vi "main.vi"() -> ()   [LabVIEW 2009]
uses:
  Support Files/VelocityState.ctl
  Support Files/TimeRec.ctl
  Support Files/LocalPose.ctl
  SimClass/Simulator.lvclass
  cRIO/Functional Global Variables/Actions for FG's.ctl
panel:
  out "Current Pose":T1={"Initial Location"={"x"=0.0, "y"=0.0}, "Initial Heading\n(degs from north)"=45.0, "Initial Location ( GPS )"={"Latitude"=0.0, "Longitude"=0.0}} {"Initial Location ( GPS )"."Longitude" format="%#_10g"; "Initial Location ( GPS )"."Latitude" format="%#_10g"}
  out "LocalPose":T2
  out "Last Yaw":dbl
  out "VelocityState":T4
  out "Current Location ( GPS )":cluster{"Latitude":dbl, "Longitude":dbl} {"Longitude" format="%#_10g"; "Latitude" format="%#_10g"}
  out "error":dbl
  in  "Loop Iteration Minimum Time":u32=100
  out "Waveform Graph":dbl[](graph)
  in  "Threshold":u32=250
  out "Turning Radius":dbl=31000000000.0
  out "Speed":dbl=133.33333333333334
  out "Compass Reading":dbl=303.2011334759296
  in  "PAUSE":bool
  out "XY Graph":cluster{dbl[], dbl[]}[](graph)=[{[35.0, 400.0, 300.0, 100.0, 300.0, 900.0, 300.0, 400.0, 500.0, 600.0, 700.0, 800.0, 200.0, 650.0, 900.0, 900.0, 800.0, 600.0], [401.0, 500.0, 0.0, 250.0, 100.0, 250.0, -400.0, 0.0, 0.0, 0.0, 0.0, 0.0, 400.0, 400.0, 400.0, 550.0, 700.0, 800.0]}, {[250.87088056783944], [819.9620618916982]}, {[250.87088056783944, 167.19553247645274], [819.9620618916982, 874.7200395916212]}, {[415.14481366760845, 410.73878540090254, 406.28405982170926, 401.781993882594, 397.23395895645433, 392.6413404187865, 388.00553722568674, 383.32796148771575, 378.6100380397561, 373.85320400699345, 369.05890836715463, 364.22861150913513, 359.3637847881498, 354.46591007754466, 349.53647931740335, 344.5769940600877, 339.58896501285085, 334.5739115776606, 329.5333613883754, 324.4688498454117, 319.38191964804645, 314.27412032449604, 309.1470077599148, 304.0021437224573, 298.84109538754876, 293.66543486050836, 288.47673869767016, 283.27658742614955, 278.0665650623987, 272.8482586297003, 267.6232576747447, 262.3931537834384, 257.15954009609175, 251.92401082213325, 246.68816075449737, 241.4535847838356, 236.221877412697, 230.99463226982752, 225.77344162473517, 220.5598959026693, 215.35558320016145, 210.16208880127624, 204.98099469471802, 199.8138790919421, 194.66231594641602, 189.5278744741782, 184.41211867583957, 179.3166068601737, 174.242891169441, 169.19251710659108, 164.1670230644875, 159.16793985729856, 154.1967902541964, 149.25508851550677, 144.3443399314505, 139.46604036361785, 134.6216757893143, 129.8127218489177, 125.04064339638354, 120.3068940530367, 115.61291576478402, 110.9601383628837, 106.34997912840475, 101.78384236050971, 97.26311894869116, 92.78918594909359, 88.36340616504867, 83.98712773195203, 79.66168370660847, 75.3883916611696, 71.16855328178877, 67.00345397211476, 62.894362461745544, 58.84253041976086, 54.84919207345166, 50.915563832362665, 47.04284391776184, 43.232211997651234, 39.484828827428146, 35.801835896307665, 32.184355079614875, 28.633488297049666, 25.15031717703215, 21.735902727227653, 18.391285011353773, 15.11748283236679, 11.915493422124541, 8.786292137619654, 5.7308321638766415, 2.7500442236024867, -0.15516370632070675, -2.983906671414104, -5.735323009167871, -8.408574611511938, -11.002847180111928, -13.517350474412183, -15.951318552350585, -18.304010003672317, -20.57470817577024, -22.762721391984428, -24.86738316229338, -26.88805238633364, -28.824113548684863, -30.674976906361906, -32.44007866845641, -34.11888116787253, -35.710873025106196, -37.21556930401573, -38.63251165953807, -39.96126847730574, -41.20143500511983, -42.35263347624249, -43.41451322446733, -44.386750790936276, -45.26905002266858, -46.06114216277109, -46.76278593230472, -47.37376760378038, -47.89390106626212, -48.32302788205874, -48.66101733498493, -48.90776647017941, -49.06320012546507, -49.12727095424492, -49.09995943992374, -48.981273901853456, -48.77125049279863, -48.46995318792426, -48.07747376530813, -47.593931777984324, -47.01947451752653, -46.354276969181, -45.59854175856486, -44.75249908994442, -43.816406676112194, -42.79054965988564, -41.675240527249514, -40.470819012169954, -39.17765199310793, -37.79613338126455, -36.32668400059214, -34.76975145960694, -33.125810015043214, -31.395360427390187, -29.57892980835561, -27.677071460302045, -25.69036470770618, -23.619414720690486, -21.46485233068256, -19.22733383825846, -16.90754081322592, -14.50617988701299, -12.023982537420181, -9.461704865805757, -6.820127366769839, -4.100054690408314, -1.3023153972081616, 1.5722382943395985, 4.522730767333968, 7.548263273185796, 10.647914205384552, 13.820739380229583, 17.06577232443655, 20.382024569535446, 23.76848595296707, 27.224124925788658, 30.747888866893675, 34.33870440365001, 37.99547773886033, 41.717094983942616, 45.50242249823208, 49.350307234298384, 53.259577089175764, 57.22904126139636, 61.25749061372028, 65.3436980414505, 69.48641884622035, 73.68439111514141, 77.93633610519373, 82.24095863274403], [1070.9881061658584, 1073.8168491309518, 1076.5682654687055, 1079.2415170710497, 1081.8357896396496, 1084.3502929339497, 1086.7842610118882, 1089.13695246321, 1091.4076506353078, 1093.5956638515222, 1095.700325621831, 1097.7209948458712, 1099.6570560082225, 1101.5079193658996, 1103.273021127994, 1104.9518236274102, 1106.5438154846438, 1108.0485117635533, 1109.4654541190757, 1110.7942109368435, 1112.0343774646576, 1113.1855759357802, 1114.247455684005, 1115.219693250474, 1116.1019924822062, 1116.8940846223086, 1117.5957283918424, 1118.206710063318, 1118.7268435257997, 1119.1559703415965, 1119.4939597945227, 1119.7407089297171, 1119.8961425850027, 1119.9602134137826, 1119.9329018994613, 1119.8142163613911, 1119.6041929523362, 1119.3028956474618, 1118.910416224846, 1118.426874237522, 1117.8524169770642, 1117.1872194287187, 1116.4314842181025, 1115.585441549482, 1114.6493491356498, 1113.6234921194232, 1112.5081829867872, 1111.3037614717077, 1110.0105944526456, 1108.6290758408022, 1107.1596264601299, 1105.6026939191447, 1103.958752474581, 1102.2283028869278, 1100.4118722678932, 1098.5100139198398, 1096.523307167244, 1094.452357180228, 1092.2977947902202, 1090.060276297796, 1087.7404832727636, 1085.3391223465505, 1082.8569249969578, 1080.2946473253435, 1077.6530698263075, 1074.932997149946, 1072.1352578567457, 1069.2607041651981, 1066.3102116922037, 1063.284679186352, 1060.1850282541532, 1057.0122030793082, 1053.767170135101, 1050.4509178900023, 1047.0644565065707, 1043.608817533749, 1040.085053592644, 1036.4942380558875, 1032.8374647206774, 1029.115847475595, 1025.3305199613055, 1021.4826352252394, 1017.5733653703619, 1013.6039011981413, 1009.5754518458173, 1005.4892444180872, 1001.3465236133172, 997.1485513443963, 992.8966063543439, 988.5919838267937, 984.2359949914672, 979.8299667247613, 975.375241145568, 970.8731752064527, 966.3251402803131, 961.7325217426453, 957.0967185495455, 952.4191428115746, 947.7012193636149, 942.9443853308522, 938.1500896910135, 933.3197928329939, 928.4549661120086, 923.5570914014035, 918.6276606412621, 913.6681753839465, 908.6801463367096, 903.6650929015195, 898.6245427122342, 893.5600311692705, 888.4731009719053, 883.3653016483548, 878.2381890837736, 873.0933250463161, 867.9322767114076, 862.7566161843672, 857.567920021529, 852.3677687500084, 847.1577463862575, 841.9394399535591, 836.7144389986036, 831.484335107297, 826.2507214199507, 821.015192145992, 815.7793420783562, 810.5447661076944, 805.3130587365558, 800.0858135936862, 794.8646229485939, 789.6510772265282, 784.4467645240202, 779.253270125135, 774.0721760185768, 768.9050604158009, 763.7534972702748, 758.619055798037, 753.5032999996984, 748.4077881840325, 743.3340724932998, 738.2836984304498, 733.2582043883464, 728.2591211811573, 723.2879715780552, 718.3462698393655, 713.4355212553093, 708.5572216874766, 703.7128571131732, 698.9039031727765, 694.1318247202423, 689.3980753768956, 684.7040970886428, 680.0513196867425, 675.4411604522635, 670.8750236843684, 666.3543002725498, 661.8803672729524, 657.4545874889075, 653.0783090558108, 648.7528650304673, 644.4795729850284, 640.2597346056475, 636.0946352959735, 631.9855437856044, 627.9337117436196, 623.9403733973105, 620.0067451562215, 616.1340252416206, 612.3233933215101, 608.5760101512868, 604.8930172201665, 601.2755364034737, 597.7246696209086, 594.2414985008909, 590.8270840510864, 587.4824663352126, 584.2086641562256, 581.0066747459833, 577.8774734614784, 574.8220134877355, 571.8412255474612]}, {[0.0, 8.258239109063283, 17.6635679516302, 28.26928085134969, 39.161034112875655, 49.351545961474756, 58.68782493571467, 67.017866895006, 74.17725616254506, 79.93157593985106, 86.00734524231453, 94.48319360575078, 105.64436487028703, 119.79167725592882, 136.94358299068747, 150.1794196360733, 164.84512081171752, 180.911713938689, 198.27358070071088, 216.77350429907193, 235.8092408864332, 255.1902209511005, 272.62384059728083, 290.25086600452346, 307.9346913572528, 325.5367474666883, 342.87942162910025, 360.2220957915122, 376.0280427586526, 391.9430716500898, 407.9108111753572, 422.5728055023587, 437.47556231438506, 452.5412559123831, 467.6519786813084, 482.6778140366067, 497.95146078225406, 513.8552236079469, 530.3377967718476, 547.0991140448708, 564.116287401357, 581.5716748487926, 599.3034974177289, 617.2698170600805, 635.4402994256407, 653.6804251256779, 671.7908807905975, 689.9856022328188, 706.4126193604907, 723.1005733700046, 739.963298873506, 756.8529674826408, 773.5504360275042, 789.8403344502048, 805.3515380864515, 819.6617215096924, 832.3140886250497, 843.200174463986, 852.4303276119743, 859.4839933491301, 863.7335964441816, 864.7675329350542, 863.7568239435701, 860.3907306643073, 854.3479289558276, 845.4083990435004, 837.0746902438183, 826.973110391912, 814.9603185789508, 800.9883210595851, 784.9800736112029, 767.0818857558896, 747.6182647298988, 732.8362291802346, 717.1776661256229, 700.7226353767547, 683.5753213617098, 665.8647841032133, 647.8264266153427, 629.7231234483743, 611.5363362750118, 596.2012632718238, 580.4652358635182, 564.408396193986, 548.1917784471037, 531.961267905226, 515.876775330523, 500.2101580493559, 485.16185522372234, 474.0051421448708, 462.8484290660192, 451.69171598716764, 440.5350029083161, 429.3782898294645, 418.22157675061294, 407.0648636717614, 395.9081505929098, 384.75143751405824, 373.5947244352067, 362.4380113563551, 351.28129827750354, 340.12458519865197, 328.9678721198004, 317.81115904094884, 306.65444596209727, 295.4977328832457, 284.34101980439414, 273.18430672554257, 262.027593646691, 250.87088056783944], [0.0, 12.328596362905685, 24.313045923484637, 35.865186506569145, 47.75528456479064, 60.89370394730574, 75.29412013383347, 90.99290161882688, 108.06433194829125, 126.50346678912352, 145.814740377611, 165.3810317097952, 184.94444001419743, 204.165762572179, 222.3316303279354, 233.66288031356822, 244.11977587242683, 253.48717156117036, 261.52322332137487, 267.99720891922806, 273.6281558953824, 278.324449702282, 280.84890240628783, 281.82999720091664, 281.24981789324136, 279.1025398162905, 275.40458966575017, 271.70663951520976, 269.7061592666714, 268.97013199980813, 268.86835635614165, 268.2364589423116, 266.480429242474, 263.5329284594952, 259.3377937103711, 253.85256193168433, 248.2881210338638, 243.92967377612416, 240.85675779555444, 237.71946831793488, 234.54566810056866, 232.8429787662082, 232.6828200848, 233.3175442229486, 233.95948113539436, 235.4416482831041, 238.60310931659052, 241.77529872967, 244.56280159826372, 248.87479650382113, 254.85314881697008, 262.63920115244434, 272.35045410822636, 284.111807811969, 297.9244947604338, 313.6561633759146, 330.9617022784776, 349.83474276684797, 371.0198243205319, 394.5080390795776, 419.86008534092036, 439.5780549826773, 460.26950127953415, 481.79548414219704, 503.8942815691288, 526.0232330481643, 541.7200682960488, 557.1819167795918, 572.2488388431018, 586.617354269714, 600.0202190589248, 612.0278146679726, 622.2118716284103, 628.2397295487174, 633.1902346453021, 636.9208635631228, 639.2929552421908, 640.1761610137296, 639.460294815211, 637.0847932487015, 634.7022118498005, 633.9962228687847, 634.4960528781803, 636.2942836022781, 639.4678027745167, 644.0782427338557, 650.1687764225292, 657.7069481835645, 666.6397243319143, 673.9407880252373, 681.2418517185604, 688.5429154118834, 695.8439791052065, 703.1450427985295, 710.4461064918526, 717.7471701851756, 725.0482338784986, 732.3492975718217, 739.6503612651447, 746.9514249584678, 754.2524886517908, 761.5535523451139, 768.8546160384369, 776.15567973176, 783.456743425083, 790.757807118406, 798.0588708117291, 805.3599345050521, 812.6609981983752, 819.9620618916982]}]
  in  "LIDAR Characteristics":T5={"Num of Sectors"=180, "Field of View (Degs)"=180.0, "Max Range"=300.0}
  in  "Obstacle Radius":dbl=30.0
  in  "Initial Vehicle Pose":T1={"Initial Location"={"x"=0.0, "y"=0.0}, "Initial Heading\n(degs from north)"=45.0, "Initial Location ( GPS )"={"Latitude"=0.0, "Longitude"=0.0}} {"Initial Location ( GPS )"."Longitude" format="%#_10g"; "Initial Location ( GPS )"."Latitude" format="%#_10g"}
  in  "stop":bool
  in  "Timestep (s)":dbl=0.1
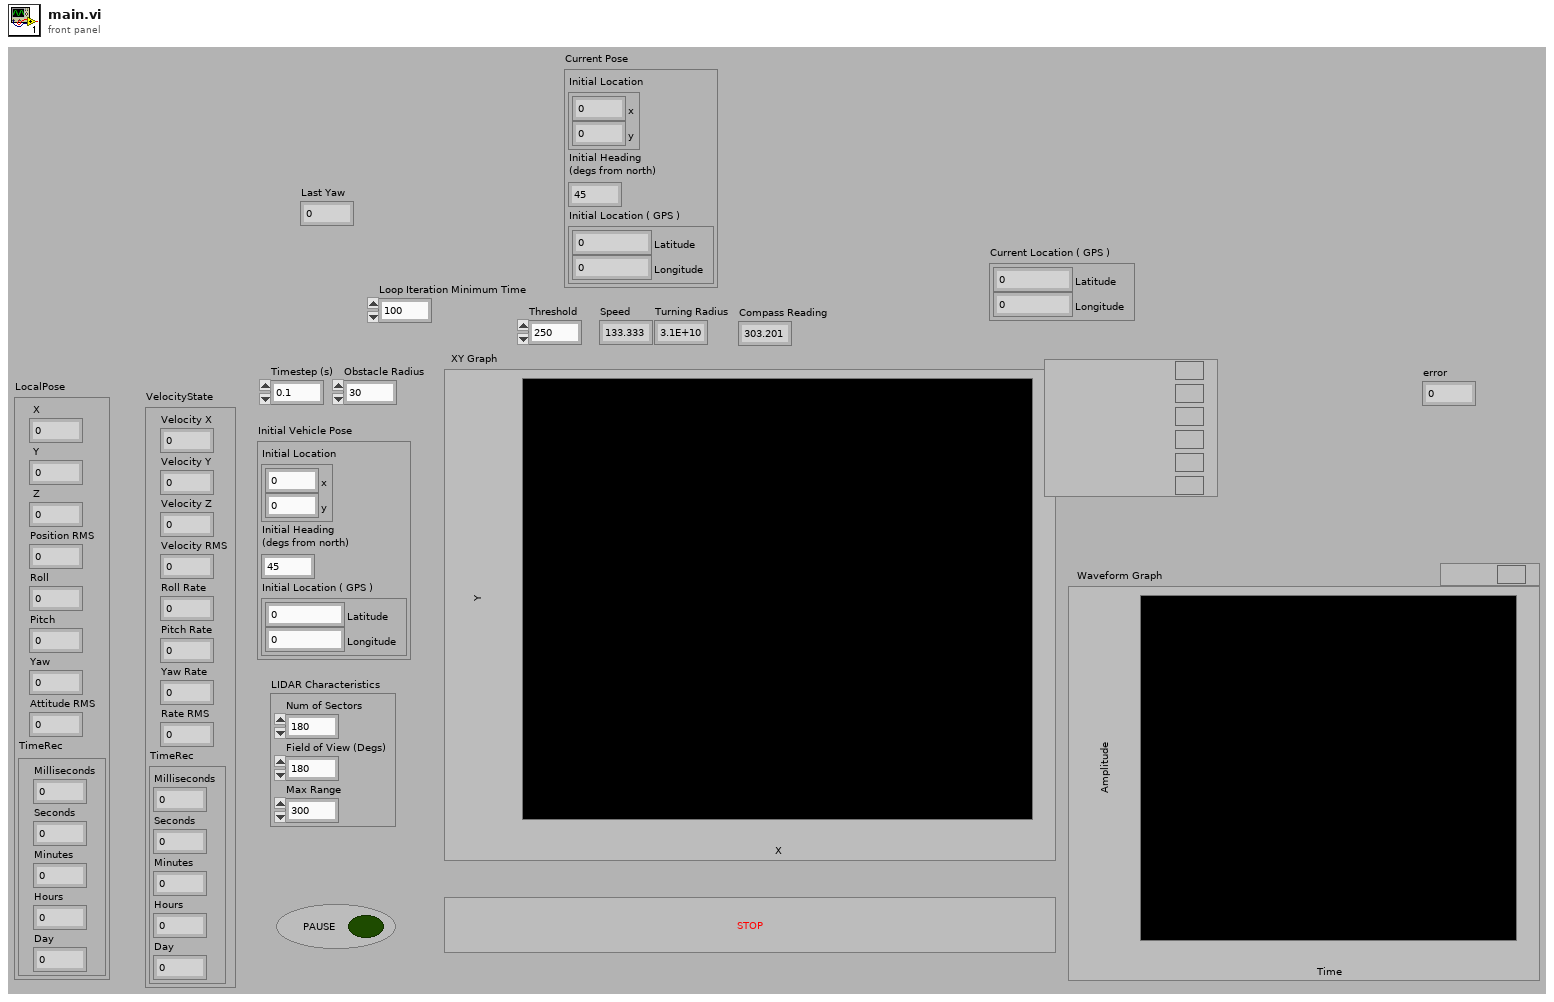
[diagram p1: front panel]
types:
  T1 = cluster{"Initial Location":cluster{"x":dbl, "y":dbl}, "Initial Heading\n(degs from north)":dbl, "Initial Location ( GPS )":cluster{"Latitude":dbl, "Longitude":dbl}}
  T2 = typedef "LocalPose.ctl" = cluster{" X":dbl, " Y":dbl, " Z":dbl, "Position RMS":dbl, "Roll":dbl, "Pitch":dbl, "Yaw":dbl, "Attitude RMS":dbl, "TimeRec":T3}
  T3 = typedef "TimeRec.ctl" = cluster{"Milliseconds":u32, "Seconds":u32, "Minutes":u32, "Hours":u32, "Day":u32}
  T4 = typedef "VelocityState.ctl" = cluster{"Velocity X":dbl, "Velocity Y":dbl, "Velocity Z":dbl, "Velocity RMS":dbl, "Roll Rate":dbl, "Pitch Rate":dbl, "Yaw Rate":dbl, "Rate RMS":dbl, "TimeRec":T3}
  T5 = cluster{"Num of Sectors":i32, "Field of View (Degs)":dbl, "Max Range":dbl}
  T6 = typedef "Actions for FG's.ctl" = enum16{"Read", "Write"}
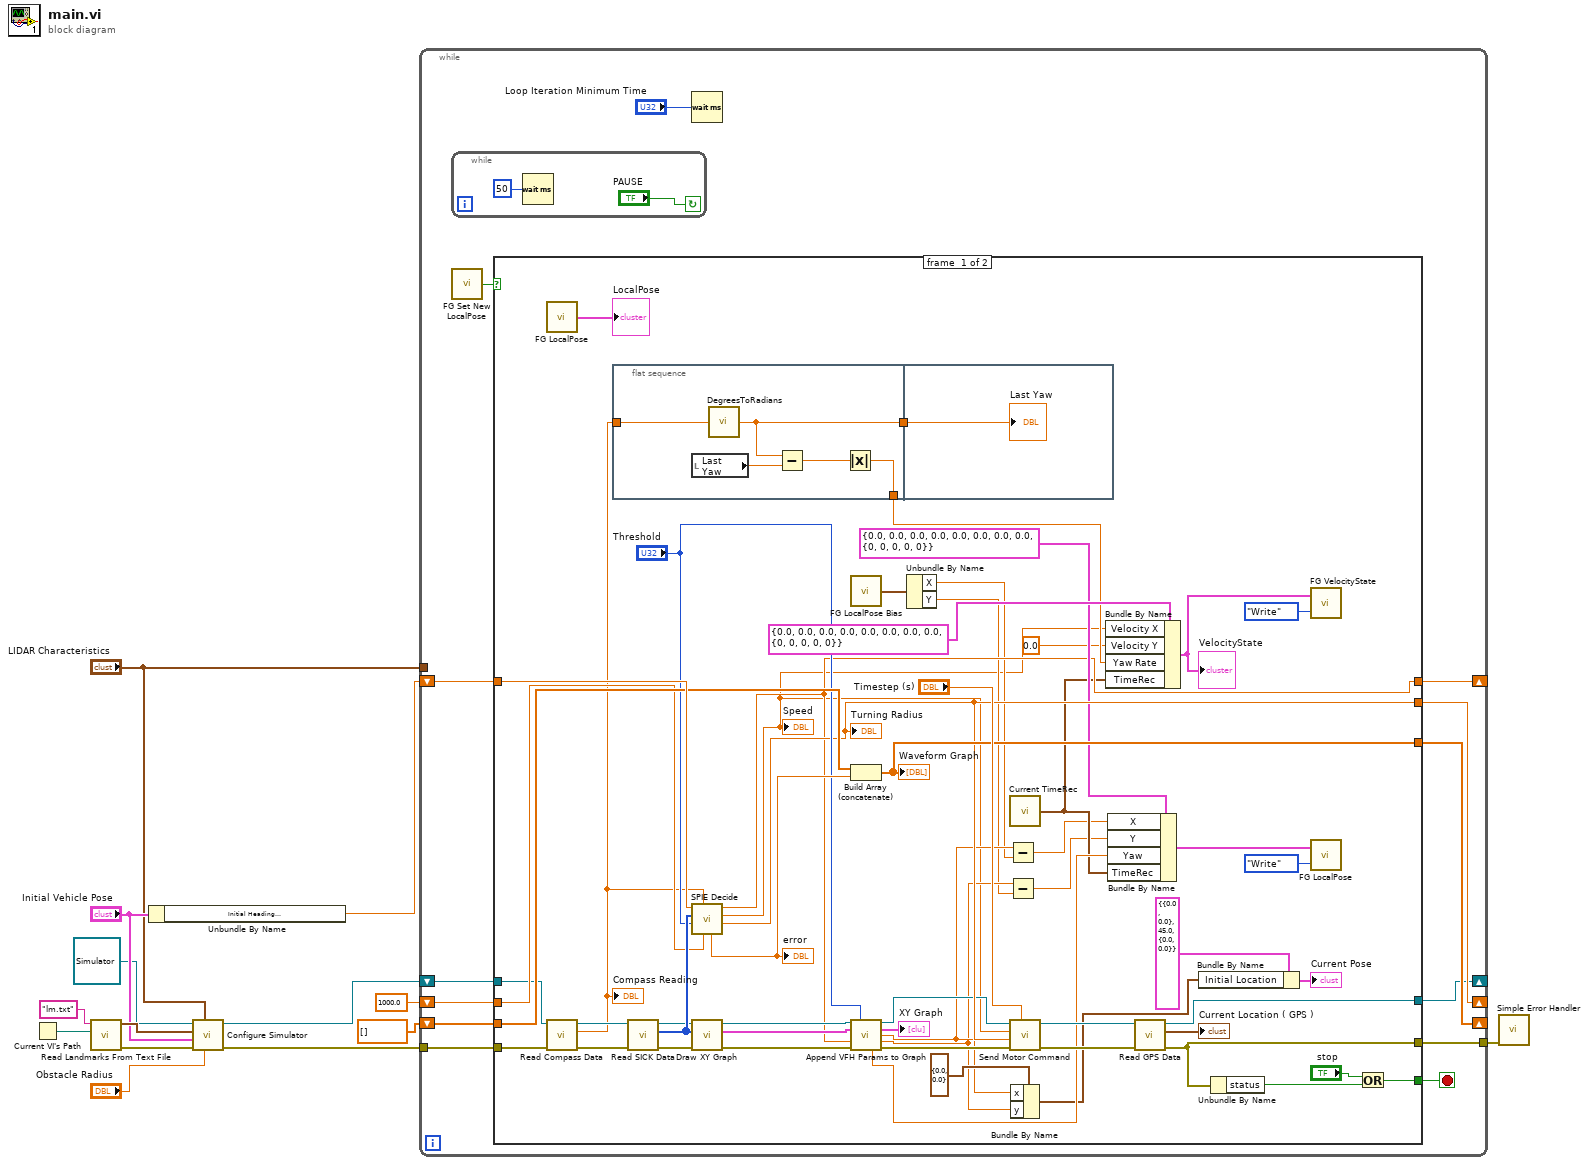
[diagram p0: block diagram]
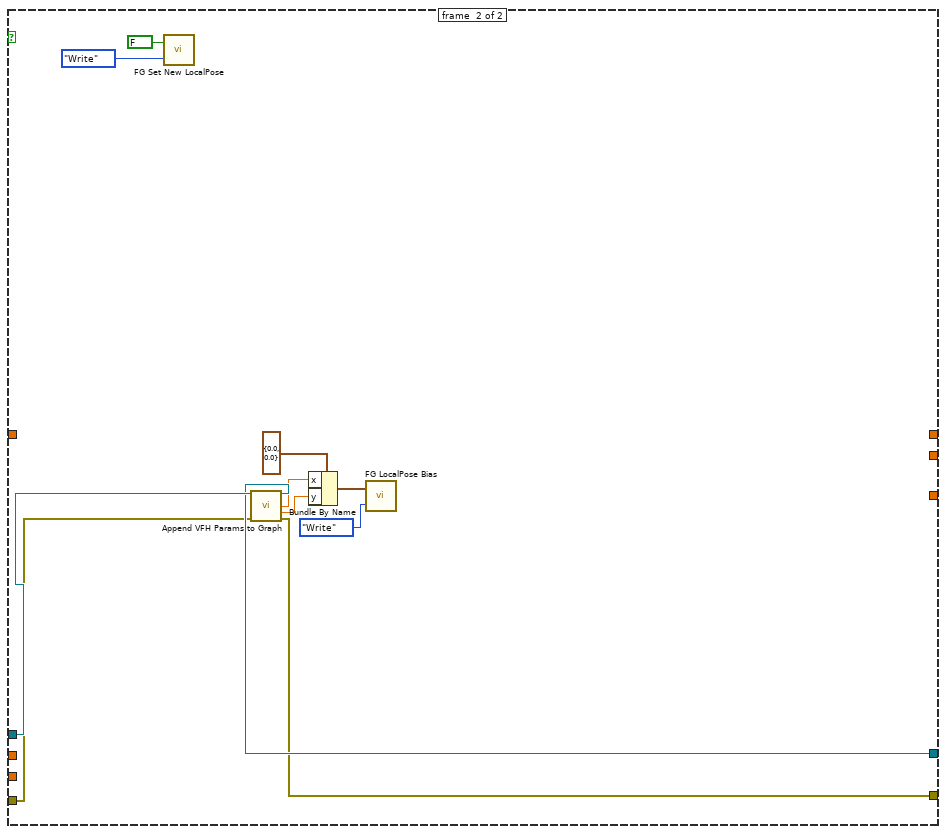
[diagram p2: hidden frame]
diagram:
  n1 = Current VI's Path() -> (path=w8:path)
  n2 = call "Read Landmarks From Text File.vi"("root VI's Path"=w8, "File Name"="lm.txt") -> ("error out"=w10:errorcluster, "Landmarks"=w11:cluster{dbl, dbl}[])  [unwired: 8 in]
  n3 = Unbundle By Name("Initial Vehicle Pose") -> ("Initial Heading\n(degs from north)"=w7:dbl)
  n4 = call-dynamic "Configure Simulator.vi"("Obstacle Radius"="Obstacle Radius", "LIDAR Characteristics"="LIDAR Characteristics", "error in (no error)"=w10, "Initial Vehicle Pose"="Initial Vehicle Pose", "Obstacle Locations"=w11, "Simulator in"=refnum<class "Simulator.lvclass"> refnum ("Simulator.lvclass")) -> ("error out"=w14:errorcluster, "Simulator out"=w1:refnum<class "Simulator.lvclass">)  [unwired: 4 in]
  n5 = while {
    tunnel: w14 -> [w24]
    shift-right: [w17] -> _
    shift-left: w1 -> [w16]
    tunnel: [w19] -> w13
    shift-right: [w18] -> _
    shift-left: w7 -> [w25]
    shift-right: [w23] -> _
    shift-left: dbl[] [] -> [w22]
    shift-right: [w20] -> _
    shift-left: 1000.0 ("Turning Radius") -> [w21]
    tunnel: "LIDAR Characteristics" -> [_]
    stop <- w27 stop-if-true
    n6 = while {
      stop <- "PAUSE" continue-if-true
      n7 = Wait (ms)(milliseconds to wait=u32 50) -> ()  [unwired: 1 out]
    }
    n8 = call "FG Set New LocalPose.vi"() -> ("Set New LocalPose Out"=w15:bool)  [unwired: 2 in]
    n9 = case shown="True" w15 {
      tunnel: [w79 _] -> w27
      tunnel: w25 -> [w76 _]
      tunnel: w24 -> [w73 w95]
      tunnel: [w72 _] -> w23
      tunnel: w22 -> [w71 _]
      tunnel: w21 -> [w67 _]
      tunnel: [w60 _] -> w20
      tunnel: [w58 w94] -> w19
      tunnel: [w46 _] -> w18
      tunnel: [w42 w96] -> w17
      tunnel: w16 -> [w37 w97]
      frame #0 {
        n10 = call "FG LocalPose.vi"() -> ("LocalPose out"=→"LocalPose":T2)  [unwired: 2 in]
        n11 = call-dynamic "Read Compass Data.vi"("error in (no error)"=w73, "Simulator in"=w37) -> ("error out"=w75:errorcluster, "Compass Reading"=w51:dbl, "Simulator out"=w74:refnum<class "Simulator.lvclass">)  [unwired: 7 in]
        "Compass Reading" <- w51
        n12 = flat-sequence {
          tunnel: w51 -> [w84]
          tunnel: [w83] -> w82
          tunnel: [w85] -> w50
          tunnel: w82 -> [w88]
          frame #0 {
            n13 = local read "Last Yaw"() -> (w87:dbl)
            n14 = call "DegreesToRadians.vi"("Degrees"=w84) -> ("Radians"=w83:dbl)
            n15 = Subtract(x=w83, y=w87) -> (x-y=w86:dbl)
            n16 = Absolute Value(x=w86) -> (abs(x)=w85:dbl)
          }
          frame #1 {
            "Last Yaw" <- w88
          }
        }
        n17 = call-dynamic "Read SICK Data.vi"("error in (no error)"=w75, "Simulator in"=w74) -> ("error out"=w68:errorcluster, "LIDAR Reading"=w77:u32[], "Simulator out"=w69:refnum<class "Simulator.lvclass">)  [unwired: 7 in]
        n18 = call "SPIE Decide.vi"("Previous Radius"=w67, "Compass Bearing_k"=w51, "Threshold"="Threshold", "SICK Data"=w77, "Decide Bearing_(k+1)"=w76) -> ("Turning Radius"=w60:dbl, "Speed"=w28:dbl, "Decide Bearing_k"=w46:dbl, "error"=w70:dbl)  [unwired: 3 in]
        "Speed" <- w28
        "Turning Radius" <- w60
        "error" <- w70
        n19 = call-dynamic "Draw XY Graph.vi"("error in (no error)"=w68, "LIDAR Scan"=w77, "Simulator in"=w69) -> ("error out"=w63:errorcluster, "XY Graph"=w65:cluster{dbl[], dbl[]}[], "Simulator out"=w64:refnum<class "Simulator.lvclass">)  [unwired: 6 in]
        n20 = call "FG LocalPose Bias.vi"() -> ("LocalPose Bias Out"=w35:cluster{"X":dbl, "Y":dbl})  [unwired: 2 in]
        n21 = Build Array (concatenate)(w71, w70) -> (w72:dbl[])
        "Waveform Graph" <- w72
        n22 = call-dynamic "Append VFH Params to Graph.vi"("Simulator in"=w64, "Threshold"="Threshold", "XY Graph in"=w65, "Calculated Bearing wrt north (degs)"=w46, "error in (no error)"=w63) -> ("Simulator out"=w55:refnum<class "Simulator.lvclass">, "XY Graph out"=→"XY Graph":cluster{dbl[], dbl[]}[], "Vehicle Location.x"=w33:dbl, "Vehicle Location.y"=w30:dbl, "Vehicle Bearing (rads)"=w48:dbl, "error out"=w62:errorcluster)  [unwired: 5 in]
        n23 = Unbundle By Name(w35) -> ("X"=w32:dbl, "Y"=w29:dbl)
        n24 = Subtract(x=w33, y=w32) -> (x-y=w34:dbl)
        n25 = Subtract(x=w30, y=w29) -> (x-y=w31:dbl)
        n26 = call "Current TimeRec.vi"() -> ("Current TimeRec"=w43:T3)
        n27 = call-dynamic "Send Motor Command.vi"("Timestep (s)"="Timestep (s)", "error in (no error)"=w62, "Turning Radius"=w60, "Speed (units/s)"=w28, "Simulator in"=w55) -> ("error out"=w59:errorcluster, "Simulator out"=w57:refnum<class "Simulator.lvclass">)  [unwired: 3 in, 2 out]
        n28 = Bundle By Name(cluster=cluster{"x":dbl, "y":dbl} {"x"=0.0, "y"=0.0} ("Initial Location"), "x"=w33, "y"=w30) -> (w39:cluster{"x":dbl, "y":dbl})
        n29 = Bundle By Name(cluster=T4 {"Velocity X"=0.0, "Velocity Y"=0.0, "Velocity Z"=0.0, "Velocity RMS"=0.0, "Roll Rate"=0.0, "Pitch Rate"=0.0, "Yaw Rate"=0.0, "Rate RMS"=0.0, "TimeRec"={"Milliseconds"=0, "Seconds"=0, "Minutes"=0, "Hours"=0, "Day"=0}} ("VelocityState"), "Velocity X"=w28, "Velocity Y"=0.0, "Yaw Rate"=w50, "TimeRec"=w43) -> (w52:T4)
        "VelocityState" <- w52
        n30 = Bundle By Name(cluster=T2 {" X"=0.0, " Y"=0.0, " Z"=0.0, "Position RMS"=0.0, "Roll"=0.0, "Pitch"=0.0, "Yaw"=0.0, "Attitude RMS"=0.0, "TimeRec"={"Milliseconds"=0, "Seconds"=0, "Minutes"=0, "Hours"=0, "Day"=0}} ("LocalPose"), "X"=w34, "Y"=w31, "Yaw"=w48, "TimeRec"=w43) -> (w44:T2)
        n31 = call-dynamic "Read GPS Data.vi"("error in (no error)"=w59, "Simulator in"=w57) -> ("error out"=w58:errorcluster, "Current Location ( GPS )"=→"Current Location ( GPS )":cluster{"Latitude":dbl, "Longitude":dbl}, "Simulator out"=w42:refnum<class "Simulator.lvclass">)  [unwired: 7 in]
        n32 = Bundle By Name(cluster=T1 {"Initial Location"={"x"=0.0, "y"=0.0}, "Initial Heading\n(degs from north)"=45.0, "Initial Location ( GPS )"={"Latitude"=0.0, "Longitude"=0.0}} ("Current Pose"), "Initial Location"=w39) -> (→"Current Pose":T1)
        n33 = Unbundle By Name(w58) -> ("status"=w78:bool)
        n34 = call "FG VelocityState.vi"("FG Action (Read)"=Actions_for_FG's."Write", "VelocityState in"=w52) -> ()  [unwired: 1 out]
        n35 = call "FG LocalPose.vi"("FG Action (Read)"=Actions_for_FG's."Write", "LocalPose in"=w44) -> ()  [unwired: 1 out]
        n36 = Or(x="stop", y=w78) -> (x .or. y?=w79:bool)
      }
      frame #1 {
        n37 = call "FG Set New LocalPose.vi"("FG Action (Read)"=Actions_for_FG's."Write", "Set New LocalPose In"=FALSE) -> ()  [unwired: 1 out]
        n38 = call-dynamic "Append VFH Params to Graph.vi"("Simulator in"=w97, "error in (no error)"=w95) -> ("Simulator out"=w96:refnum<class "Simulator.lvclass">, "Vehicle Location.x"=w90:dbl, "Vehicle Location.y"=w89:dbl, "error out"=w94:errorcluster)  [unwired: 8 in, 2 out]
        n39 = Bundle By Name(cluster=cluster{"x":dbl, "y":dbl} {"x"=0.0, "y"=0.0} ("Initial Location"), "x"=w90, "y"=w89) -> (w91:cluster{"x":dbl, "y":dbl})
        n40 = call "FG LocalPose Bias.vi"("FG Action (Read)"=Actions_for_FG's."Write", "LocalPose Bias In"=w91) -> ()  [unwired: 1 out]
      }
    }
    n41 = Wait (ms)(milliseconds to wait="Loop Iteration Minimum Time") -> ()  [unwired: 1 out]
  }
  n42 = call <vilib>:"Simple Error Handler.vi"("error in (no error)"=w13) -> ()  [unwired: 4 in, 5 out]
